vi "Initialise.vi"(8 "error in (no error)":errorcluster, 10 "Instrument Ref":string, 11 "Chroma190020 HiPOT in":refnum<class "Chroma190020 HiPOT.lvclass">) -> (0 "error out":errorcluster, 3 "Chroma190020 HiPOT out":refnum<class "Chroma190020 HiPOT.lvclass">)   [LabVIEW 2019, in "Concrete.lvlib" / "Chroma190020 HiPOT.lvclass"]
uses:
  Chroma190020 HiPOT.lvclass
  Chroma190020 HiPOT.lvclass/Chroma190020 HiPOT.ctl
  Harware Abstraction/Analog In/Analog In.lvclass
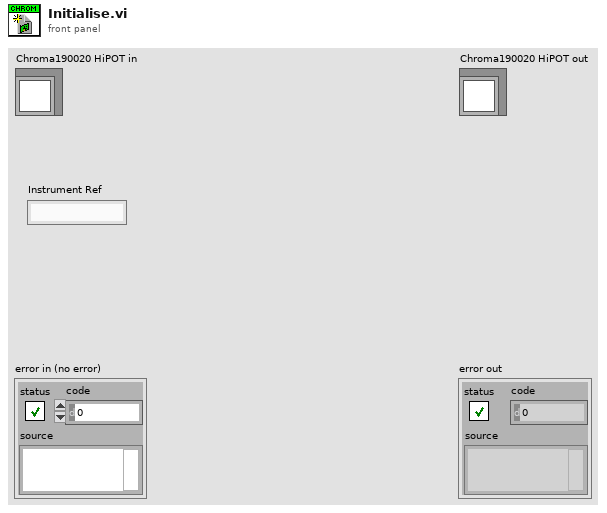
[diagram p1: front panel]
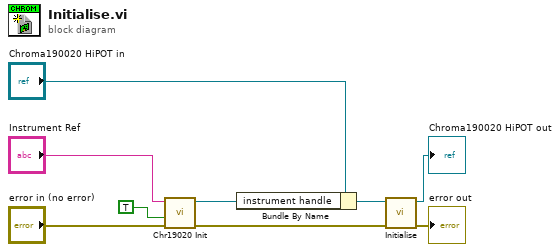
[diagram p0: block diagram]
diagram:
  n1 = call <instrlib>:"Chr19020 Init.vi"("error in (no error)"="error in (no error)", "reset device"=TRUE, "resource name"="Instrument Ref") -> ("error out"=w5:errorcluster, "instrument handle out"=w1:refnum<k15>)  [unwired: 7 in]
  n2 = Bundle By Name(cluster="Chroma190020 HiPOT in", "instrument handle"=w1) -> (w2:refnum<class "Chroma190020 HiPOT.lvclass">)
  n3 = call-parent "Initialise.vi"("error in (no error)"=w5, "Instrument in"=w2) -> ("error out"=→"error out":errorcluster, "Instrument out"=→"Chroma190020 HiPOT out":refnum<class "Chroma190020 HiPOT.lvclass">)  [unwired: 8 in]
